vi "wifi-init_com.vi"(6 "timeout (10sec)":u32=10000, 8 "error in (no error)":errorcluster, 10 "port":u32, 11 "IP address":refnum<visa-resource-name>="COM13") -> (0 "error out":errorcluster)   [LabVIEW 2023, in "wifi-interface.lvlib"]
uses:
  wifi-interface.lvlib
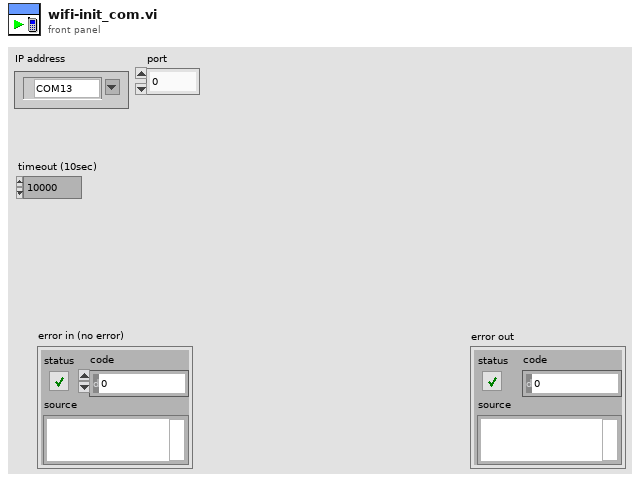
[diagram p1: front panel]
types:
  T1 = enum16{"init", "broadcast_data", "receive_data", "close", "clear_visa"}
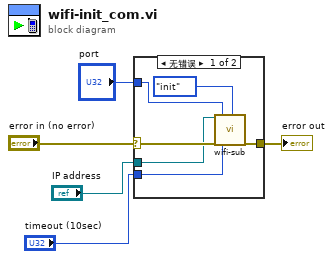
[diagram p0: block diagram]
diagram:
  n1 = case shown="无错误" "error in (no error)" {
    selector: "error in (no error)" -> [w10 w12]
    tunnel: [w11 w12] -> w4
    tunnel: "IP address" -> [w6 _]
    tunnel: "timeout (10sec)" -> [w7 _]
    tunnel: "port" -> [w9 _]
    frame No Error {
      n2 = call "wifi-sub.vi"("IP address"=w6, "error in (no error)"=w10, "port"=w9, "timeout (10sec)"=w7, "mode"=T1."init") -> ("error IO"=w11:errorcluster)  [unwired: 13 in, 1 out]
    }
    frame Error {
    }
  }
  "error out" <- w4
